vi "Drive Core.vi"(0 "A Encoder BL":string="My Motor RefNum", 1 "Rotational Motor FR":string="My Motor RefNum", 2 "Rotational Motor FL":string="My Motor RefNum", 3 "Rotational Motor BR":string="My Motor RefNum", 4 "Rotational Motor BL":string="My Motor RefNum", 5 "Drive Motor FR":string="My Motor RefNum", 6 "A Encoder BR":string="My Motor RefNum", 7 "Drive Motor FL":string="My Motor RefNum", 8 "A Encoder FL":string="My Motor RefNum", 9 "Drive Motor BR":string="My Motor RefNum", 10 "A Encoder FR":string="My Motor RefNum", 11 "Drive Motor BL":string="My Motor RefNum", 12 "Enabled?":bool=TRUE) -> ()   [LabVIEW 2012]
uses:
  Begin/Global Variables.vi
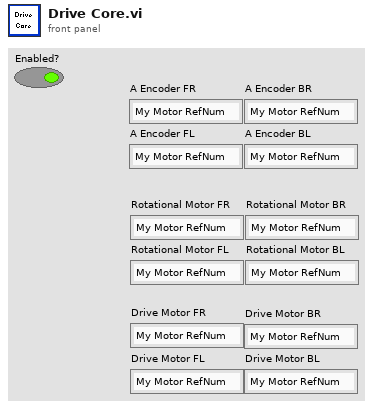
[diagram p1: front panel]
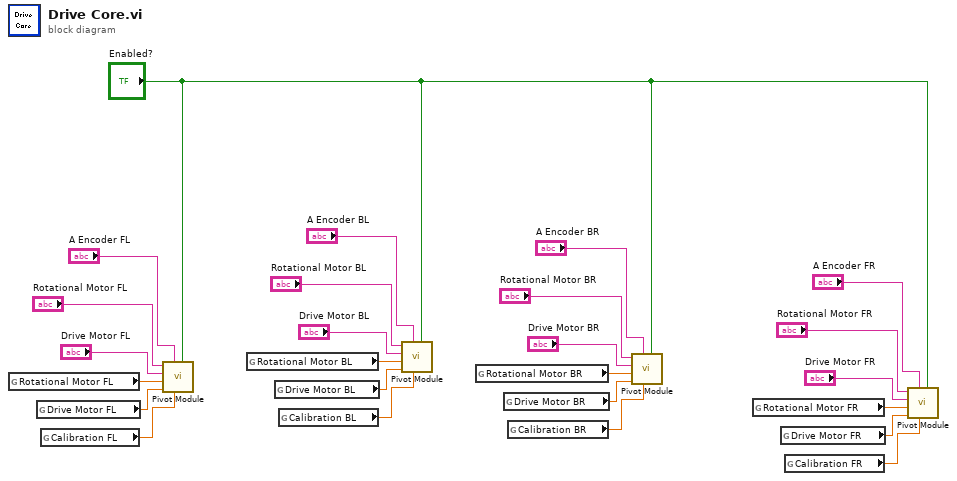
[diagram p0: block diagram]
diagram:
  n1 = global read "Global Variables.vi" "Rotational Motor FL"() -> (w4:dbl)
  n2 = global read "Global Variables.vi" "Drive Motor FL"() -> (w14:dbl)
  n3 = global read "Global Variables.vi" "Calibration FL"() -> (w5:dbl)
  n4 = call "Pivot Module.vi"("Boolean"="Enabled?", "Calibration Angle"=w5, "Encoder Refnum"="A Encoder FL", "Motor Speed"=w14, "Motor Angle"=w4, "Drive Motor Refnum"="Drive Motor FL", "Rotational Motor Refnum"="Rotational Motor FL") -> ()  [unwired: 5 in]
  n5 = global read "Global Variables.vi" "Rotational Motor BL"() -> (w2:dbl)
  n6 = global read "Global Variables.vi" "Drive Motor BL"() -> (w16:dbl)
  n7 = global read "Global Variables.vi" "Calibration BL"() -> (w7:dbl)
  n8 = call "Pivot Module.vi"("Boolean"="Enabled?", "Calibration Angle"=w7, "Encoder Refnum"="A Encoder BL", "Motor Speed"=w16, "Motor Angle"=w2, "Drive Motor Refnum"="Drive Motor BL", "Rotational Motor Refnum"="Rotational Motor BL") -> ()  [unwired: 5 in]
  n9 = global read "Global Variables.vi" "Rotational Motor BR"() -> (w3:dbl)
  n10 = global read "Global Variables.vi" "Drive Motor BR"() -> (w15:dbl)
  n11 = global read "Global Variables.vi" "Calibration BR"() -> (w6:dbl)
  n12 = call "Pivot Module.vi"("Boolean"="Enabled?", "Calibration Angle"=w6, "Encoder Refnum"="A Encoder BR", "Motor Speed"=w15, "Motor Angle"=w3, "Drive Motor Refnum"="Drive Motor BR", "Rotational Motor Refnum"="Rotational Motor BR") -> ()  [unwired: 5 in]
  n13 = global read "Global Variables.vi" "Rotational Motor FR"() -> (w22:dbl)
  n14 = global read "Global Variables.vi" "Drive Motor FR"() -> (w21:dbl)
  n15 = global read "Global Variables.vi" "Calibration FR"() -> (w20:dbl)
  n16 = call "Pivot Module.vi"("Boolean"="Enabled?", "Calibration Angle"=w20, "Encoder Refnum"="A Encoder FR", "Motor Speed"=w21, "Motor Angle"=w22, "Drive Motor Refnum"="Drive Motor FR", "Rotational Motor Refnum"="Rotational Motor FR") -> ()  [unwired: 5 in]
